vi "AbortMultiple.vi"(8 "error in (no error)":errorcluster, 10 "axis names":string[](array[string]), 11 "controller in":refnum<k24>) -> (0 "error out":errorcluster, 3 "controller out":refnum<k24>)   [LabVIEW 2013]
uses:
  C:/GEECS/Developers Version/source/Device Driver/AerotechStage/Sample Vis/Bin/Aerotech.Ensemble.dll
  Bin/Aerotech.Ensemble.dll
  C:/GEECS/Developers Version/source/Device Driver/AerotechStage/Sample Vis/Bin/Aerotech.Ensemble.LabVIEW.dll
  Bin/Aerotech.Ensemble.LabVIEW.dll
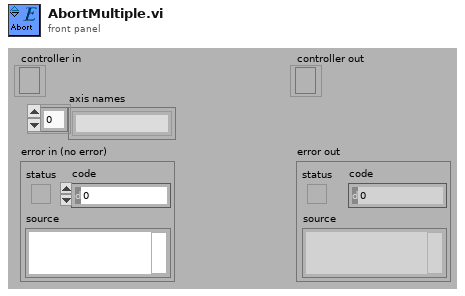
[diagram p1: front panel]
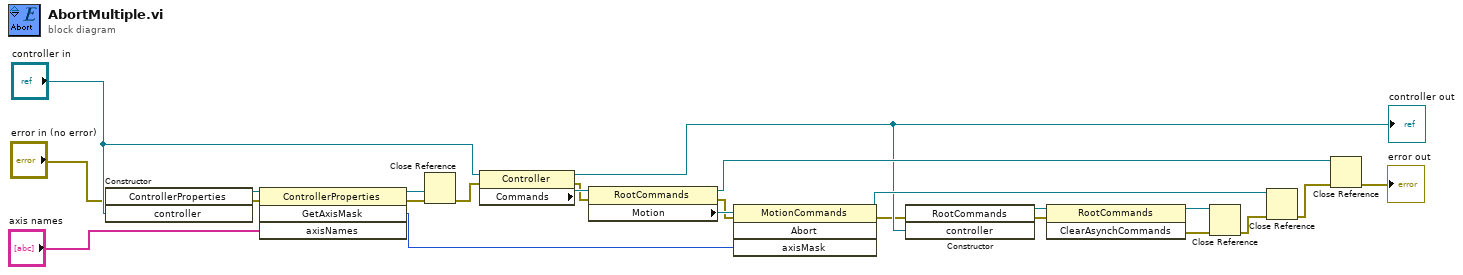
[diagram p0: block diagram]
diagram:
  n1 = constructor class="ControllerProperties"(error in="error in (no error)", "controller"="controller in") -> (reference out=w15:refnum<k24>, error out=w14:errorcluster)  [unwired: 2 in, 2 out]
  n2 = invoke class="ControllerProperties" method="GetAxisMask"(reference=w15, error in=w14, "axisNames"="axis names") -> (reference out=w12:refnum<k24>, error out=w13:errorcluster, "GetAxisMask"=w10:i32)  [unwired: 1 in, 1 out]
  n3 = Close Reference(reference=w12, error in (no error)=w13) -> (error out=w11:errorcluster)
  n4 = property class="Controller"(reference="controller in", error in=w11) -> (reference out=w2:refnum<k24>, error out=w22:errorcluster, "Commands"=w24:refnum<k24>)
  "controller out" <- w2
  n5 = property class="RootCommands"(reference=w24, error in=w22) -> (reference out=w17:refnum<k24>, error out=w21:errorcluster, "Motion"=w23:refnum<k24>)
  n6 = invoke class="MotionCommands" method="Abort"(reference=w23, error in=w21, "axisMask"=w10) -> (reference out=w18:refnum<k24>, error out=w1:errorcluster)  [unwired: 1 in, 2 out]
  n7 = constructor class="RootCommands"(error in=w1, "controller"=w2) -> (reference out=w7:refnum<k24>, error out=w4:errorcluster)  [unwired: 2 in, 2 out]
  n8 = invoke class="RootCommands" method="ClearAsynchCommands"(reference=w7, error in=w4) -> (reference out=w5:refnum<k24>, error out=w6:errorcluster)  [unwired: 1 in, 1 out]
  n9 = Close Reference(reference=w5, error in (no error)=w6) -> (error out=w3:errorcluster)
  n10 = Close Reference(reference=w18, error in (no error)=w3) -> (error out=w19:errorcluster)
  n11 = Close Reference(reference=w17, error in (no error)=w19) -> (error out=→"error out":errorcluster)
